vi "ReadData.vi"(8 "error in (no error)":errorcluster, 11 "NI_DAQmx(Linear) in":refnum<class "NI_DAQmx(Linear).lvclass">) -> (0 "error out":errorcluster, 2 "Waveform":waveform(dbl)[](array[waveform]), 3 "NI_DAQmx(Linear) out":refnum<class "NI_DAQmx(Linear).lvclass">)   [LabVIEW 2025, in "NI_DAQmx(Linear).lvclass"]
uses:
  NI_DAQmx(Linear).lvclass
  NI_DAQmx(Linear).lvclass/NI_DAQmx(Linear).ctl
  <vilib>/DAQmx/read.llb/DAQmx Read (Counter 2D DBL NChan NSamp).vi
  Read task.vi
  <vilib>/DAQmx/miscellaneous.llb/DAQmx Fill In Error Info.vi
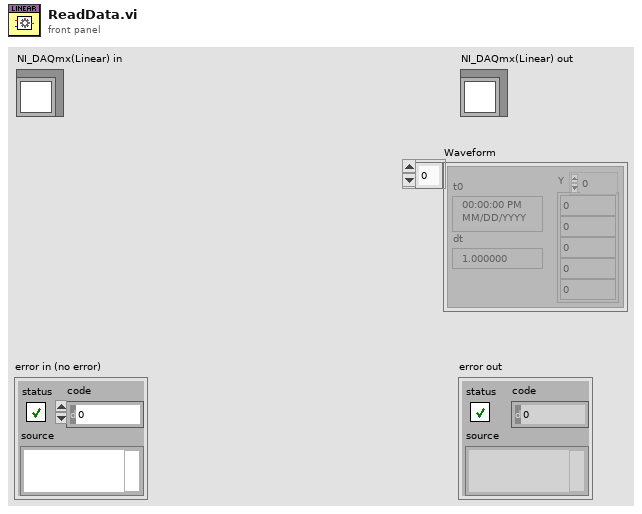
[diagram p1: front panel]
types:
  T1 = typedef "DAQ_Module.lvlib/DAQ_Module.lvclass/DAQ_Task_Config.ctl" = cluster{"Drive":T2, "TaskType":T3, "PhysicalChannels":string, "SampleRateConfiguration":T4, "ChannelConfig":map{string, cluster{"PhysicalChannels":string, "Config":string}}, "Enable":bool, "ShowPanel":bool}
  T2 = typedef "DAQ_Module.lvlib/DAQ_Module.lvclass/DAQ_HW_Type.ctl" = enum16{"NI_DAQmx", "Simulated_DAQ"}
  T3 = typedef "DAQ_Module.lvlib/DAQ_Module.lvclass/DAQ_Task_Type.ctl" = enum16{"AI", "Linear", "Angular", "AO"}
  T4 = typedef "DAQ_Module.lvlib/DAQ_Module.lvclass/DAQ_SampleRateConfig.ctl" = cluster{"SampleRate":dbl, "SamplesPerChannel":u32, "SamplesPerRead":i32, "SampleMode":i32, "Clock Source":string}
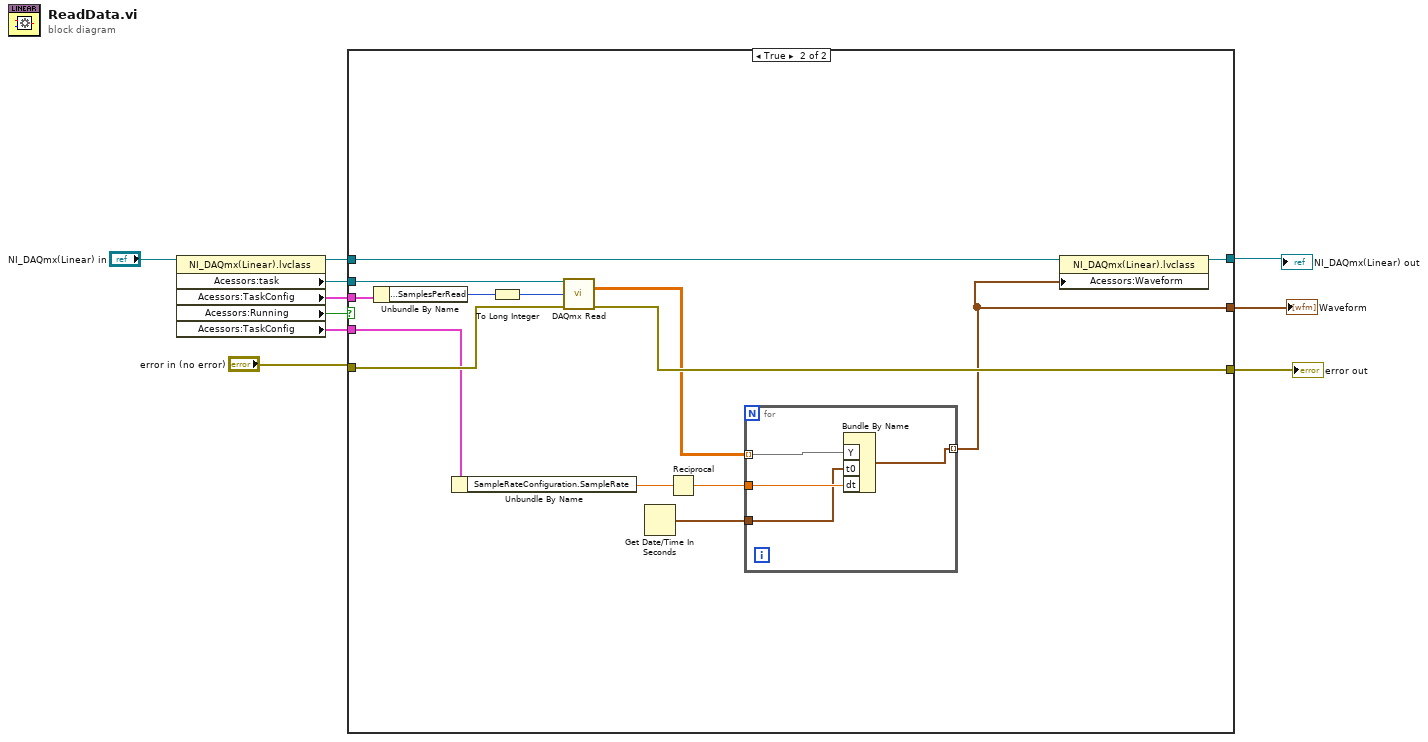
[diagram p0: block diagram]
diagram:
  n1 = property class="NI_DAQmx(Linear).lvclass"(reference="NI_DAQmx(Linear) in") -> (reference out=w8:refnum<class "NI_DAQmx(Linear).lvclass">, "Acessors:task"=w10:refnum<k21>, "Acessors:TaskConfig"=w9:T1, "Acessors:Running"=w7:bool, "Acessors:TaskConfig"=w1:T1)  [unwired: 1 in, 1 out]
  n2 = case shown="True" w7 {
    tunnel: w10 -> [_ w13]
    tunnel: "error in (no error)" -> [w11 w26]
    tunnel: [w11 w25] -> w3
    tunnel: w9 -> [_ w24]
    tunnel: w8 -> [w12 w21]
    tunnel: [w12 w20] -> w5
    tunnel: [_ w18] -> w2
    tunnel: w1 -> [_ w17]
    frame False {
    }
    frame True {
      n3 = Unbundle By Name(w24) -> ("SampleRateConfiguration.SamplesPerRead"=w23:i32)
      n4 = Unbundle By Name(w17) -> ("SampleRateConfiguration.SampleRate"=w16:dbl)
      n5 = To Long Integer(number=w23) -> (32bit integer=w22:i32)
      n6 = call-poly <vilib>:"DAQmx Read.vi"("task/channels in"=w13, "number of samples per channel"=w22, "error in"=w26) -> ("data"=w19:dbl[][], "error out"=w25:errorcluster)  [unwired: 10 in, 1 out]
      n7 = Get Date/Time In Seconds() -> (seconds since 1Jan1904=w14:timestamp)
      n8 = Reciprocal(x=w16) -> (1/x=w15:dbl)
      n9 = for {
        tunnel: w19 -> [w30] mode=indexing
        tunnel: [w29] -> w18 mode=indexing
        tunnel: w15 -> [w28]
        tunnel: w14 -> [w27]
        n10 = Bundle By Name("Y"=w30, "t0"=w27, "dt"=w28) -> (w29:waveform(dbl))  [unwired: 1 in]
      }
      n11 = property class="NI_DAQmx(Linear).lvclass"(reference=w21, "Acessors:Waveform"=w18) -> (reference out=w20:refnum<class "NI_DAQmx(Linear).lvclass">)  [unwired: 1 in, 1 out]
    }
  }
  "error out" <- w3
  "NI_DAQmx(Linear) out" <- w5
  "Waveform" <- w2
